vi "HTVacuumGUI.constructor.vi"(0 "name":string, 2 "data in":string, 5 "error in (no error)":errorcluster) -> (14 "i ref out":refnum<vi>, 16 "data out":string, 19 "error out":errorcluster)   [LabVIEW 2014, in "HTVacuumGUI.lvlib"]
doc: "This is the constructor of a class.\n\nLicense Agreement for this software:\n\nCopyright (C)\nGesellschaft für Schwerionenforschung, GSI\nPlanckstr. 1\n64291 Darmstadt\nGermany\n\nContact: D.Beck@gsi.de \n\nThis program is free software; you can redistribute it and/or modify it under the terms of the \nGNU General Public License as published by the Free Software Foundation; either version 2 of \nthe license, or (at your option) any later version.\n\nThis program is distributed in the hope that it will be useful, but WITHOUT ANY WARRANTY; \nwithout even the implied warranty of MERCHANTABILITY or FITNESS FOR A PARTICULAR PURPOSE. See the GNU General License for more details (http://www.gnu.org).\n\nGesellschaft für Schwerionenforschung, GSI\nPlanckstr. 1, 64291 Darmstadt, Germany\nFor all questions and ideas contact: M.Richter@gsi.de, H.Brand@gsi.de or D.Beck@gsi.de.\nLast update: 16-JUN-2004"
uses:
  HTVacuumGUI.lvlib
  CSCore/CSSystem/CSSystemLib/CSSystemLib.lvlib
  CSCore/GUIs/GOGUserGUIs/DeviceBaseGUI/DeviceBaseGUI.lvlib
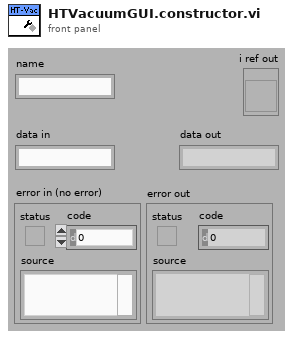
[diagram p1: front panel]
types:
  T1 = enum16{"SetAttribute", "GetAttribute", "CreateAttribute", "DestroyAttribute", "DestroyAllAtributes"}
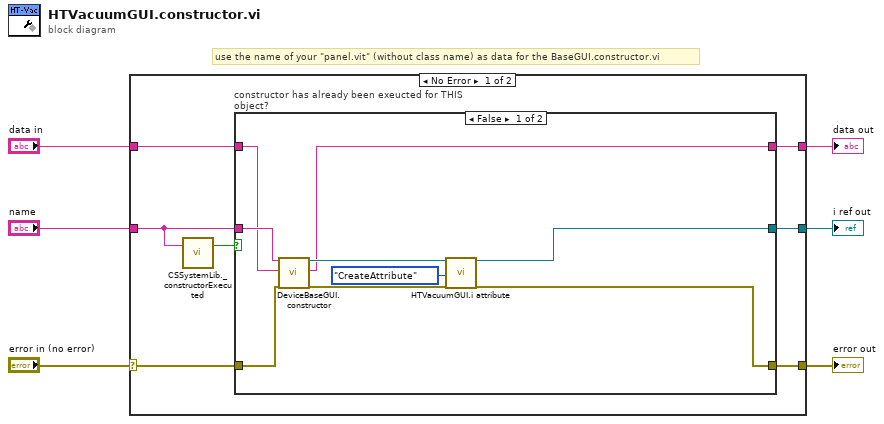
[diagram p0: block diagram]
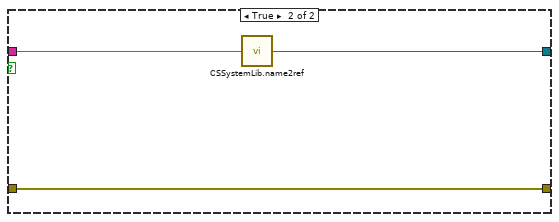
[diagram p2: hidden frame]
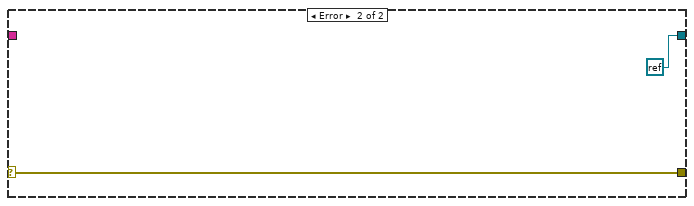
[diagram p3: hidden frame]
diagram:
  # "use the name of your \"panel.vit\" (without class name) as data for the BaseGUI.constructor.vi"
  n1 = case shown="No Error" "error in (no error)" {
    selector: "error in (no error)" -> [w10 w26]
    tunnel: "data in" -> [w13 _]
    tunnel: "name" -> [w9 _]
    tunnel: [w12 refnum<k0> refnum] -> w4
    tunnel: [w11 w26] -> w3
    tunnel: [w7 _] -> w1
    frame No Error {
      n2 = call "CSSystemLib._constructorExecuted.vi"("name"=w9) -> ("constructor executed?"=w8:bool)  [unwired: 18 in]
      n3 = case "constructor has already been exeucted for THIS object?" shown="False" w8 {
        tunnel: w13 -> [w15 _]
        tunnel: w9 -> [w17 w25]
        tunnel: [w21 w24] -> w12
        tunnel: [w16 w23] -> w11
        tunnel: w10 -> [w20 w23]
        tunnel: [w14 _] -> w7
        frame False {
          n4 = call "DeviceBaseGUI.constructor.vi"("name"=w17, "data in"=w15, "error in (no error)"=w20) -> ("i ref out"=w18:refnum<vi>, "data out"=w14:string, "error out"=w19:errorcluster)  [unwired: 14 in]
          n5 = call "HTVacuumGUI.i attribute.vi"("VI Refnum"=w18, "Action"=T1."CreateAttribute", "error in (no error)"=w19) -> ("VI Refnum out"=w21:refnum<vi>, "error out"=w16:errorcluster)  [unwired: 14 in, 1 out]
        }
        frame True {
          n6 = call "CSSystemLib.name2ref.vi"("name"=w25) -> ("obj refnum"=w24:refnum<vi>)
        }
      }
    }
    frame Error {
    }
  }
  "i ref out" <- w4
  "error out" <- w3
  "data out" <- w1
